vi "manageActiveTestModuleRef.vi"(8 "error in (no error)":errorcluster, 10 "operation":enum16{"read", "update"}(ring), 11 "New TestModule Ref":refnum<vi>) -> (0 "error out":errorcluster, 3 "ActiveTestModule Ref":refnum<vi>)   [LabVIEW 2015, in "pdbm_task_route.lvlib"]
uses:
  pdbm_task_route.lvlib
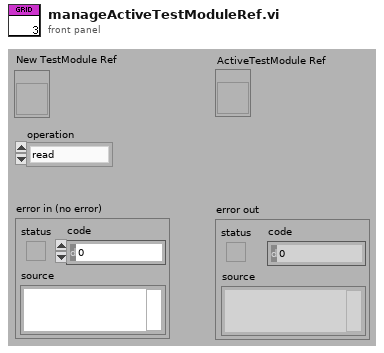
[diagram p1: front panel]
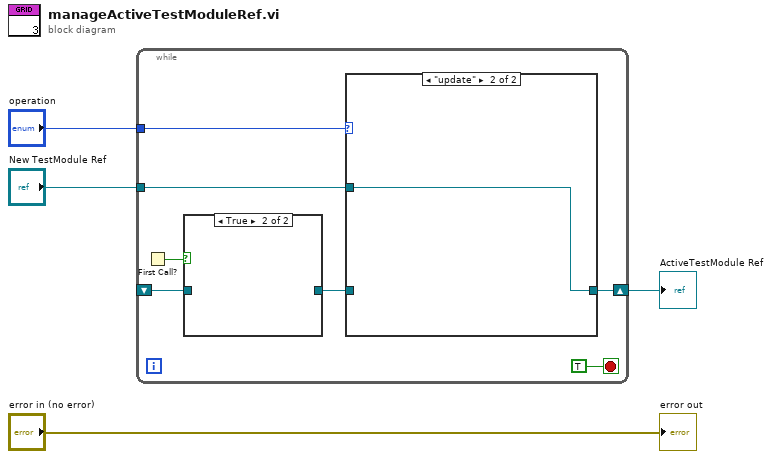
[diagram p0: block diagram]
diagram:
  n1 = while {
    tunnel: "operation" -> [w8]
    shift-right: [w6] -> w2
    shift-left: _ -> [w9]
    tunnel: "New TestModule Ref" -> [w5]
    stop <- TRUE stop-if-true
    n2 = First Call?() -> (First Call?: T/F=w10:bool)
    n3 = case shown="True" w10 {
      tunnel: w9 -> [w14 _]
      tunnel: [w14 _] -> w7
      frame False {
      }
      frame True {
      }
    }
    n4 = case shown="\"update\"" w8 {
      tunnel: w7 -> [w12 _]
      tunnel: [w12 w13] -> w6
      tunnel: w5 -> [_ w13]
      frame "read", Default {
      }
      frame "update" {
      }
    }
  }
  "ActiveTestModule Ref" <- w2
  "error out" <- "error in (no error)"
